vi "configFileReader.vi"(1 "error (in)":errorcluster, 2 "file (use dialog)":path) -> (0 "error (out)":errorcluster)   [LabVIEW 2016]
doc: "Grab the .project8_authentications.json file in the home and read the AMQP credentials."
uses:
  global/Config_Infos.vi
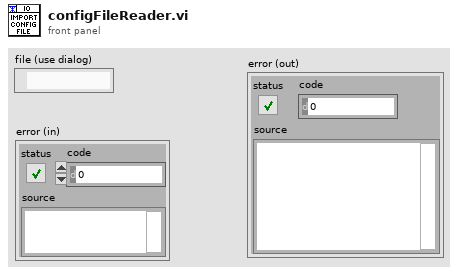
[diagram p1: front panel]
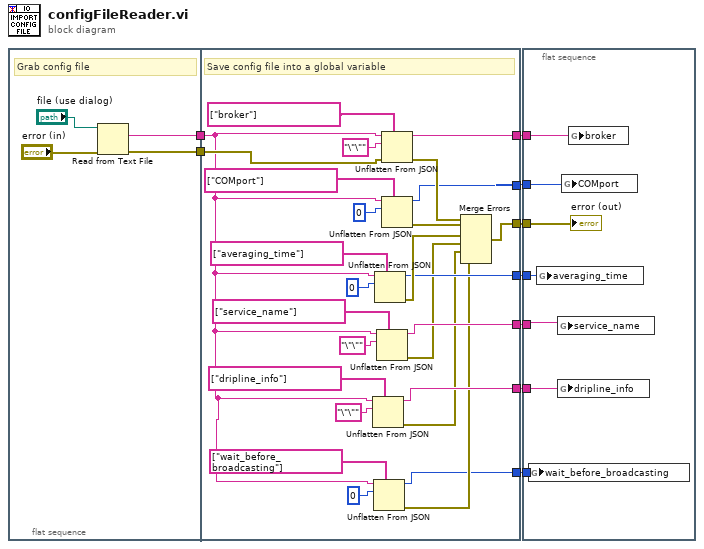
[diagram p0: block diagram]
diagram:
  n1 = flat-sequence {
    tunnel: [w13] -> w9
    tunnel: [w12] -> w8
    tunnel: w9 -> [w16]
    tunnel: w8 -> [w38]
    tunnel: [w35] -> w5
    tunnel: [w34] -> w7
    tunnel: [w33] -> w6
    tunnel: [w29] -> w4
    tunnel: [w24] -> w3
    tunnel: [w20] -> w2
    tunnel: [w14] -> w1
    frame #0 {
      # "Grab config file"
      n2 = Read from Text File(file (use dialog)="file (use dialog)", error in="error (in)") -> (text=w13:string, error out=w12:errorcluster)  [unwired: 2 in, 2 out]
    }
    frame #1 {
      # "Save config file into a global variable"
      n3 = Unflatten From JSON(path=string[] ["dripline_info"], JSON string=w16, type and defaults="\"\"") -> (value=w20:string, error out=w19:errorcluster)  [unwired: 4 in]
      n4 = Unflatten From JSON(path=string[] ["wait_before_broadcasting"], JSON string=w16, type and defaults=0) -> (value=w14:i32, error out=w15:errorcluster)  [unwired: 4 in]
      n5 = Unflatten From JSON(path=string[] ["averaging_time"], JSON string=w16, type and defaults=0) -> (value=w29:i32, error out=w30:errorcluster)  [unwired: 4 in]
      n6 = Unflatten From JSON(path=string[] ["service_name"], JSON string=w16, type and defaults="\"\"") -> (value=w24:string, error out=w23:errorcluster)  [unwired: 4 in]
      n7 = Unflatten From JSON(path=string[] ["broker"], JSON string=w16, type and defaults="\"\"", error in (no error)=w38) -> (value=w34:string, error out=w37:errorcluster)  [unwired: 3 in]
      n8 = Unflatten From JSON(path=string[] ["COMport"], JSON string=w16, type and defaults=0) -> (value=w33:i32, error out=w36:errorcluster)  [unwired: 4 in]
      n9 = Merge Errors(w37, w36, w30, w23, w19, w15) -> (w35:errorcluster)
    }
  }
  n10 = flat-sequence {
    tunnel: w7 -> [w47]
    tunnel: w6 -> [w46]
    tunnel: w5 -> [w45]
    tunnel: w4 -> [w44]
    tunnel: w3 -> [w43]
    tunnel: w2 -> [w42]
    tunnel: w1 -> [w41]
    frame #0 {
      n11 = global write "Config_Infos.vi" "wait_before_broadcasting"(w41) -> ()
      n12 = global write "Config_Infos.vi" "averaging_time"(w44) -> ()
      n13 = global write "Config_Infos.vi" "service_name"(w43) -> ()
      n14 = global write "Config_Infos.vi" "dripline_info"(w42) -> ()
      n15 = global write "Config_Infos.vi" "COMport"(w46) -> ()
      n16 = global write "Config_Infos.vi" "broker"(w47) -> ()
      "error (out)" <- w45
    }
  }
